vi "getSenMshape.vi"(8 "error in (no error)":errorcluster, 10 "Sen M File Name":string="senM_35_19_50.txt", 11 "OptStateEsti in":refnum<class "OptStateEsti.lvclass">) -> (0 "error out":errorcluster, 2 "Sensitivity Matrix Shape":T1={"Num of Field"=35, "Num of Zk"=19, "Num of DOF"=50}, 3 "OptStateEsti out":refnum<class "OptStateEsti.lvclass">)   [LabVIEW 2016, in "OfcFunc.lvlib" / "OptStateEsti.lvclass"]
doc: "Get the shape of sensitivity matrix M, which should be a 3D array."
uses:
  OptStateEsti.lvclass
  <vilib>/regexp/Match Regular Expression.xnode
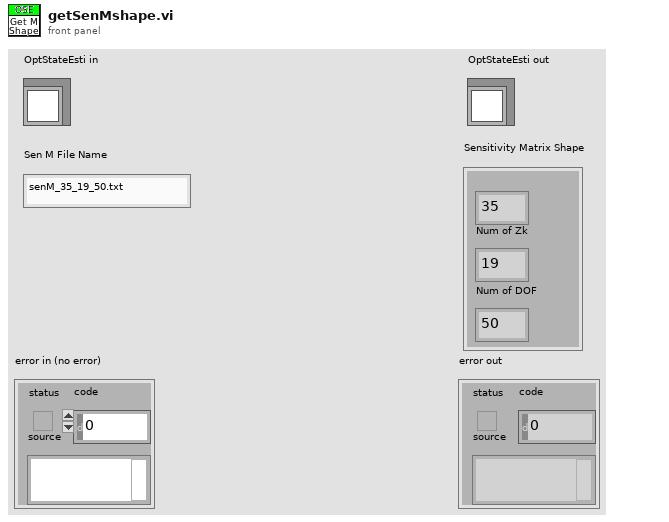
[diagram p1: front panel]
types:
  T1 = cluster{"Num of Field":i32, "Num of Zk":i32, "Num of DOF":i32}
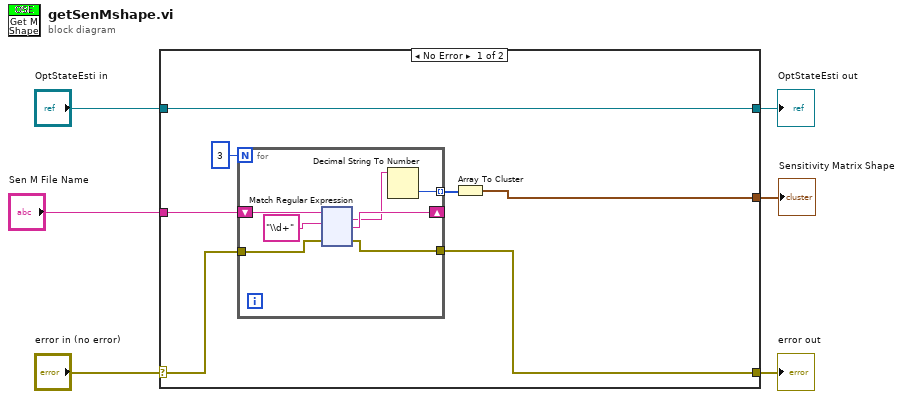
[diagram p0: block diagram]
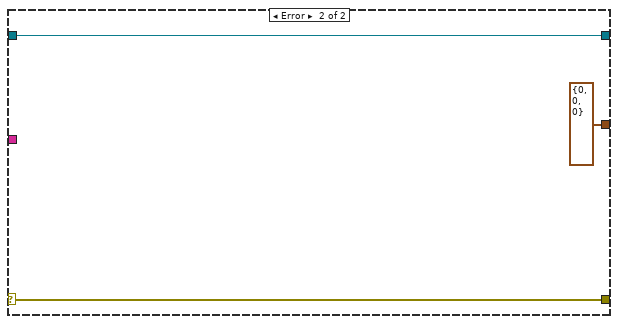
[diagram p2: hidden frame]
diagram:
  n1 = case shown="No Error" "error in (no error)" {
    selector: "error in (no error)" -> [w9 w137]
    tunnel: [w8 w137] -> w5
    tunnel: [w13 w136] -> w3
    tunnel: "OptStateEsti in" -> [w13 w136]
    tunnel: "Sen M File Name" -> [w10 _]
    tunnel: [w7 cluster{"[0]":i32, "[1]":i32, "[2]":i32} {"[0]"=0, "[1]"=0, "[2]"=0}] -> w1
    frame No Error {
      n2 = for {
        N: 3 -> [_]
        shift-right: [w18] -> _
        shift-left: w10 -> [w19]
        tunnel: [w16] -> w11 mode=indexing
        tunnel: w9 -> [w15]
        tunnel: [w14] -> w8
        n3 = xnode "Match Regular Expression"("input string"=w19, "regular expression"="\\d+", "error in"=w15) -> ("whole match"=w17:string, "after match"=w18:string, "error out"=w14:errorcluster)  [unwired: 3 in, 2 out]
        n4 = Decimal String To Number(string=w17) -> (number=w16:i32)  [unwired: 2 in, 1 out]
      }
      n5 = Array To Cluster(array=w11) -> (cluster=w7:cluster{"[0]":i32, "[1]":i32, "[2]":i32})
    }
    frame Error {
    }
  }
  "error out" <- w5
  "OptStateEsti out" <- w3
  "Sensitivity Matrix Shape" <- w1
